vi "ArdnoChannel2Valves.vi"(1 "Channel":u32, 3 "error in (no error)":errorcluster) -> (7 "Valve Nums":i32[](array[numeric]), 8 "Valve State":bool[](array[boolean]), 10 "error out":errorcluster)   [LabVIEW 2018]
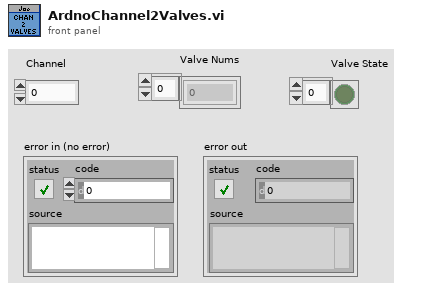
[diagram p1: front panel]
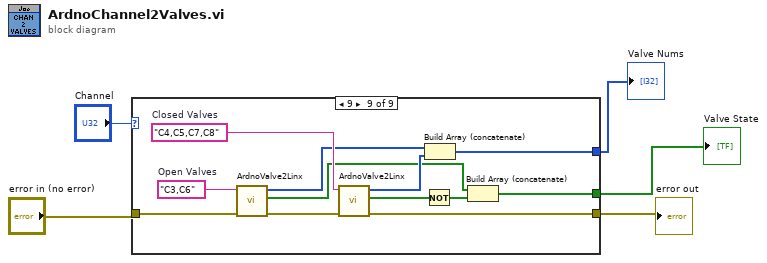
[diagram p0: block diagram]
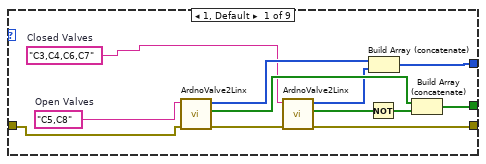
[diagram p2: hidden frame]
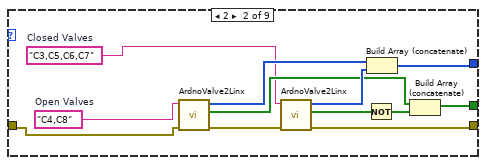
[diagram p3: hidden frame]
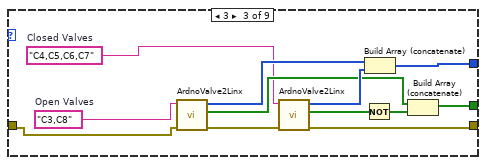
[diagram p4: hidden frame]
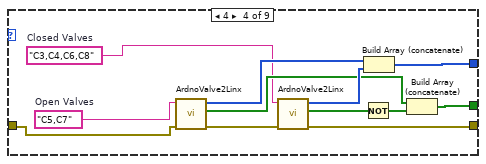
[diagram p5: hidden frame]
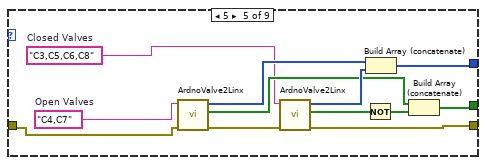
[diagram p6: hidden frame]
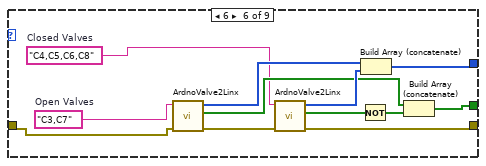
[diagram p7: hidden frame]
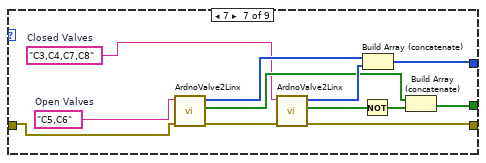
[diagram p8: hidden frame]
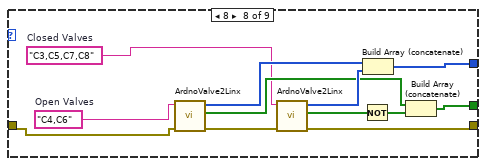
[diagram p9: hidden frame]
diagram:
  n1 = case shown="9" "Channel" {
    tunnel: [w6 w18 w35 w47 w59 w66 w83 w95 w108] -> w1
    tunnel: [w7 w20 w33 w45 w57 w68 w81 w93 w104] -> w3
    tunnel: [w11 w19 w34 w46 w58 w67 w82 w94 w103] -> w2
    tunnel: "error in (no error)" -> [w8 w21 w30 w42 w56 w69 w79 w91 w102]
    frame 1, Default {
      w10 = "C3,C4,C6,C7"  # Closed Valves
      w9 = "C5,C8"  # Open Valves
      n2 = call "ArdnoValve2Linx.vi"("error in (no error)"=w8, "Valve (A1-C8),\n comma separated"=w9) -> ("error out"=w17:errorcluster, "Closed State"=w15:bool[], "Linx Port"=w14:i32[])  [unwired: 7 in]
      n3 = call "ArdnoValve2Linx.vi"("error in (no error)"=w17, "Valve (A1-C8),\n comma separated"=w10) -> ("error out"=w7:errorcluster, "Closed State"=w12:bool[], "Linx Port"=w13:i32[])  [unwired: 7 in]
      n4 = Not(x=w12) -> (.not. x?=w16:bool[])
      n5 = Build Array (concatenate)(w14, w13) -> (w6:i32[])
      n6 = Build Array (concatenate)(w15, w16) -> (w11:bool[])
    }
    frame 2 {
      w23 = "C3,C5,C6,C7"  # Closed Valves
      w22 = "C4,C8"  # Open Valves
      n7 = call "ArdnoValve2Linx.vi"("error in (no error)"=w21, "Valve (A1-C8),\n comma separated"=w22) -> ("error out"=w24:errorcluster, "Closed State"=w26:bool[], "Linx Port"=w27:i32[])  [unwired: 7 in]
      n8 = call "ArdnoValve2Linx.vi"("error in (no error)"=w24, "Valve (A1-C8),\n comma separated"=w23) -> ("error out"=w20:errorcluster, "Closed State"=w29:bool[], "Linx Port"=w28:i32[])  [unwired: 7 in]
      n9 = Not(x=w29) -> (.not. x?=w25:bool[])
      n10 = Build Array (concatenate)(w27, w28) -> (w18:i32[])
      n11 = Build Array (concatenate)(w26, w25) -> (w19:bool[])
    }
    frame 3 {
      w32 = "C4,C5,C6,C7"  # Closed Valves
      w31 = "C3,C8"  # Open Valves
      n12 = call "ArdnoValve2Linx.vi"("error in (no error)"=w30, "Valve (A1-C8),\n comma separated"=w31) -> ("error out"=w36:errorcluster, "Closed State"=w38:bool[], "Linx Port"=w39:i32[])  [unwired: 7 in]
      n13 = call "ArdnoValve2Linx.vi"("error in (no error)"=w36, "Valve (A1-C8),\n comma separated"=w32) -> ("error out"=w33:errorcluster, "Closed State"=w41:bool[], "Linx Port"=w40:i32[])  [unwired: 7 in]
      n14 = Not(x=w41) -> (.not. x?=w37:bool[])
      n15 = Build Array (concatenate)(w39, w40) -> (w35:i32[])
      n16 = Build Array (concatenate)(w38, w37) -> (w34:bool[])
    }
    frame 4 {
      w43 = "C3,C4,C6,C8"  # Closed Valves
      w44 = "C5,C7"  # Open Valves
      n17 = call "ArdnoValve2Linx.vi"("error in (no error)"=w42, "Valve (A1-C8),\n comma separated"=w44) -> ("error out"=w48:errorcluster, "Closed State"=w50:bool[], "Linx Port"=w51:i32[])  [unwired: 7 in]
      n18 = call "ArdnoValve2Linx.vi"("error in (no error)"=w48, "Valve (A1-C8),\n comma separated"=w43) -> ("error out"=w45:errorcluster, "Closed State"=w53:bool[], "Linx Port"=w52:i32[])  [unwired: 7 in]
      n19 = Not(x=w53) -> (.not. x?=w49:bool[])
      n20 = Build Array (concatenate)(w51, w52) -> (w47:i32[])
      n21 = Build Array (concatenate)(w50, w49) -> (w46:bool[])
    }
    frame 5 {
      w54 = "C3,C5,C6,C8"  # Closed Valves
      w55 = "C4,C7"  # Open Valves
      n22 = call "ArdnoValve2Linx.vi"("error in (no error)"=w56, "Valve (A1-C8),\n comma separated"=w55) -> ("error out"=w60:errorcluster, "Closed State"=w62:bool[], "Linx Port"=w63:i32[])  [unwired: 7 in]
      n23 = call "ArdnoValve2Linx.vi"("error in (no error)"=w60, "Valve (A1-C8),\n comma separated"=w54) -> ("error out"=w57:errorcluster, "Closed State"=w65:bool[], "Linx Port"=w64:i32[])  [unwired: 7 in]
      n24 = Not(x=w65) -> (.not. x?=w61:bool[])
      n25 = Build Array (concatenate)(w63, w64) -> (w59:i32[])
      n26 = Build Array (concatenate)(w62, w61) -> (w58:bool[])
    }
    frame 6 {
      w71 = "C4,C5,C6,C8"  # Closed Valves
      w70 = "C3,C7"  # Open Valves
      n27 = call "ArdnoValve2Linx.vi"("error in (no error)"=w69, "Valve (A1-C8),\n comma separated"=w70) -> ("error out"=w72:errorcluster, "Closed State"=w74:bool[], "Linx Port"=w75:i32[])  [unwired: 7 in]
      n28 = call "ArdnoValve2Linx.vi"("error in (no error)"=w72, "Valve (A1-C8),\n comma separated"=w71) -> ("error out"=w68:errorcluster, "Closed State"=w77:bool[], "Linx Port"=w76:i32[])  [unwired: 7 in]
      n29 = Not(x=w77) -> (.not. x?=w73:bool[])
      n30 = Build Array (concatenate)(w75, w76) -> (w66:i32[])
      n31 = Build Array (concatenate)(w74, w73) -> (w67:bool[])
    }
    frame 7 {
      w78 = "C3,C4,C7,C8"  # Closed Valves
      w80 = "C5,C6"  # Open Valves
      n32 = call "ArdnoValve2Linx.vi"("error in (no error)"=w79, "Valve (A1-C8),\n comma separated"=w80) -> ("error out"=w84:errorcluster, "Closed State"=w86:bool[], "Linx Port"=w87:i32[])  [unwired: 7 in]
      n33 = call "ArdnoValve2Linx.vi"("error in (no error)"=w84, "Valve (A1-C8),\n comma separated"=w78) -> ("error out"=w81:errorcluster, "Closed State"=w89:bool[], "Linx Port"=w88:i32[])  [unwired: 7 in]
      n34 = Not(x=w89) -> (.not. x?=w85:bool[])
      n35 = Build Array (concatenate)(w87, w88) -> (w83:i32[])
      n36 = Build Array (concatenate)(w86, w85) -> (w82:bool[])
    }
    frame 8 {
      w90 = "C3,C5,C7,C8"  # Closed Valves
      w92 = "C4,C6"  # Open Valves
      n37 = call "ArdnoValve2Linx.vi"("error in (no error)"=w91, "Valve (A1-C8),\n comma separated"=w92) -> ("error out"=w96:errorcluster, "Closed State"=w98:bool[], "Linx Port"=w99:i32[])  [unwired: 7 in]
      n38 = call "ArdnoValve2Linx.vi"("error in (no error)"=w96, "Valve (A1-C8),\n comma separated"=w90) -> ("error out"=w93:errorcluster, "Closed State"=w101:bool[], "Linx Port"=w100:i32[])  [unwired: 7 in]
      n39 = Not(x=w101) -> (.not. x?=w97:bool[])
      n40 = Build Array (concatenate)(w99, w100) -> (w95:i32[])
      n41 = Build Array (concatenate)(w98, w97) -> (w94:bool[])
    }
    frame 9 {
      w112 = "C4,C5,C7,C8"  # Closed Valves
      w113 = "C3,C6"  # Open Valves
      n42 = call "ArdnoValve2Linx.vi"("error in (no error)"=w102, "Valve (A1-C8),\n comma separated"=w113) -> ("error out"=w105:errorcluster, "Closed State"=w107:bool[], "Linx Port"=w109:i32[])  [unwired: 7 in]
      n43 = call "ArdnoValve2Linx.vi"("error in (no error)"=w105, "Valve (A1-C8),\n comma separated"=w112) -> ("error out"=w104:errorcluster, "Closed State"=w111:bool[], "Linx Port"=w110:i32[])  [unwired: 7 in]
      n44 = Not(x=w111) -> (.not. x?=w106:bool[])
      n45 = Build Array (concatenate)(w109, w110) -> (w108:i32[])
      n46 = Build Array (concatenate)(w107, w106) -> (w103:bool[])
    }
  }
  "error out" <- w3
  "Valve Nums" <- w1
  "Valve State" <- w2
